vi "LVClass_WavefrontCorrector Assert User Prefs and Move to Absolute Position.vi"(0 "WavefrontCorrector in":refnum<class "WavefrontCorrector.lvclass">, 2 "Check position before move":bool, 5 "Wavefront Corrector State":T2[](array[typedef]), 7 "Sleep after command apply (ms)":i32, 9 "Position":T1, 11 "error in (no error)":errorcluster) -> (4 "WavefrontCorrector out":refnum<class "WavefrontCorrector.lvclass">, 15 "error out":errorcluster)   [LabVIEW 2020, in "WavefrontCorrector.lvclass"]
uses:
  WavefrontCorrector.lvclass
  Controls/Wavefront Corrector states - ONE.ctl
  Controls/Wavefront Corrector Position.ctl
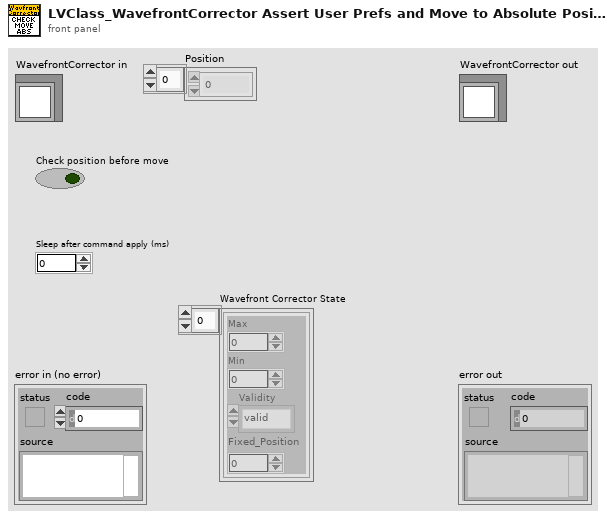
[diagram p1: front panel]
types:
  T1 = typedef "Wavefront Corrector Position.ctl" = sgl[]
  T2 = typedef "Wavefront Corrector states - ONE.ctl" = cluster{"Max":sgl, "Min":sgl, "Validity":enum16{"valid", "fixed", "invalid"}, "Fixed_Position":sgl}
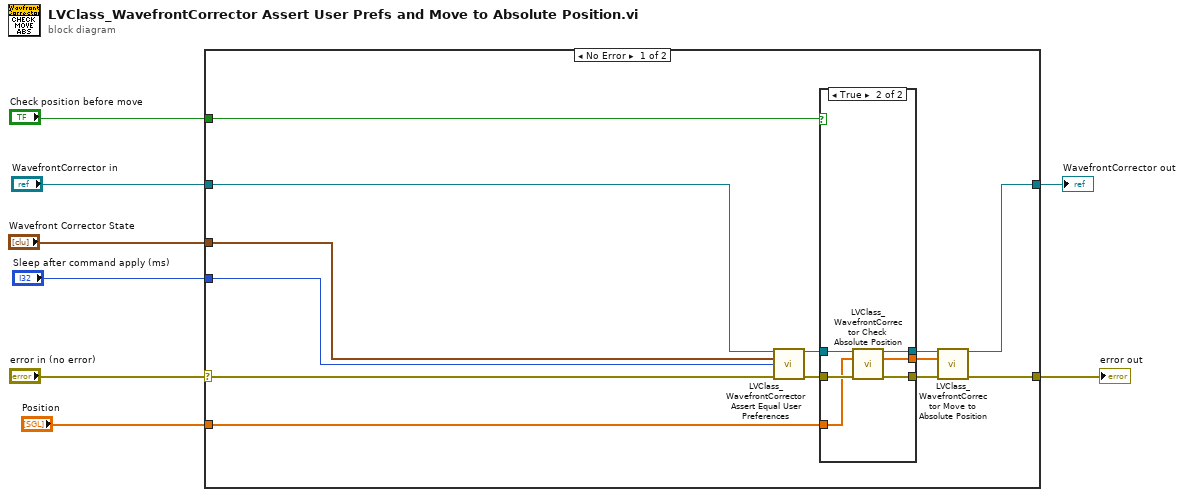
[diagram p0: block diagram]
diagram:
  n1 = case shown="No Error" "error in (no error)" {
    selector: "error in (no error)" -> [w16 w32]
    tunnel: [w19 w32] -> w5
    tunnel: [w9 w31] -> w6
    tunnel: "WavefrontCorrector in" -> [w13 w31]
    tunnel: "Check position before move" -> [w14 _]
    tunnel: "Wavefront Corrector State" -> [w12 _]
    tunnel: "Sleep after command apply (ms)" -> [w11 _]
    tunnel: "Position" -> [w10 _]
    frame No Error {
      n2 = call "LVClass_WavefrontCorrector Assert Equal User Preferences.vi"("WavefrontCorrector in"=w13, "Wavefront Corrector State"=w12, "Sleep after command apply (ms)"=w11, "error in (no error)"=w16) -> ("WavefrontCorrector out"=w17:refnum<class "WavefrontCorrector.lvclass">, "error out"=w15:errorcluster)  [unwired: 10 in]
      n3 = case shown="True" w14 {
        tunnel: [w23 w30] -> w21
        tunnel: [w22 w29] -> w20
        tunnel: [w24 w28] -> w18
        tunnel: w17 -> [w23 w27]
        tunnel: w15 -> [w22 w26]
        tunnel: w10 -> [w24 w25]
        frame False {
        }
        frame True {
          n4 = call "LVClass_WavefrontCorrector Check Absolute Position.vi"("WavefrontCorrector in"=w27, "Absolute Positions"=w25, "error in (no error)"=w26) -> ("WavefrontCorrector out"=w30:refnum<class "WavefrontCorrector.lvclass">, "Absolute Positions OUT"=w28:T1, "error out"=w29:errorcluster)  [unwired: 10 in]
        }
      }
      n5 = call "LVClass_WavefrontCorrector Move to Absolute Position.vi"("WavefrontCorrector in"=w21, "Absolute Positions"=w18, "error in (no error)"=w20) -> ("WavefrontCorrector out"=w9:refnum<class "WavefrontCorrector.lvclass">, "error out"=w19:errorcluster)  [unwired: 11 in]
    }
    frame Error {
    }
  }
  "error out" <- w5
  "WavefrontCorrector out" <- w6
